vi "PicamParameter Enum From Label.vi"(11 "String":string) -> (0 "error out":errorcluster, 3 "Numeric":i32)   [LabVIEW 2020, in "Dashboard.lvlib"]
uses:
  Dashboard.lvlib
  f4b859da-84c7-4f49-914b-b007c7d86b52.vi
  Camera/Camera.lvlib
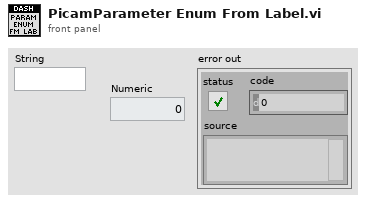
[diagram p1: front panel]
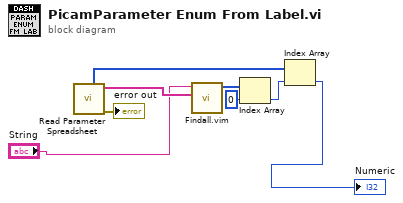
[diagram p0: block diagram]
diagram:
  n1 = call "Read Parameter Spreadsheet.vi"() -> ("error out"=→"error out":errorcluster, "Names"=w3:string[], "EnumVals"=w7:i32[])  [unwired: 7 in, 2 out]
  n2 = call "Findall.vim"("Array"=w3, "String"="String") -> ("Array"=w4:i32[])  [unwired: 9 in]
  n3 = Index Array(array=w4, index=0) -> (element=w6:i32)
  n4 = Index Array(array=w7, index=w6) -> (element=→"Numeric":i32)
